vi "SHA-2_hash chunk_U32.vi"(0 "h in":u32[](array[numeric]), 1 "Chunk":u32[](array[numeric]), 12 "error in (no error)":errorcluster) -> (4 "h out":u32[](array[numeric]), 14 "error out":errorcluster)   [LabVIEW 2011, in "i3-external-encryption.lvlib"]
doc: "Hashes a U32 chunk.\n\n(c) Ton Plomp, 2011\nTHIS SOFTWARE IS PROVIDED AS IS, AND ANY WARRANTY IS REJECTED"
uses:
  i3-external-encryption.lvlib
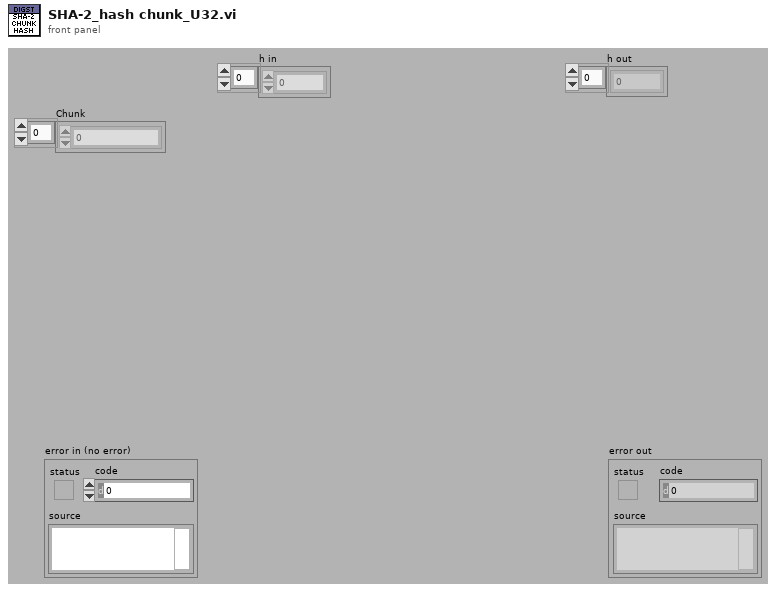
[diagram p1: front panel]
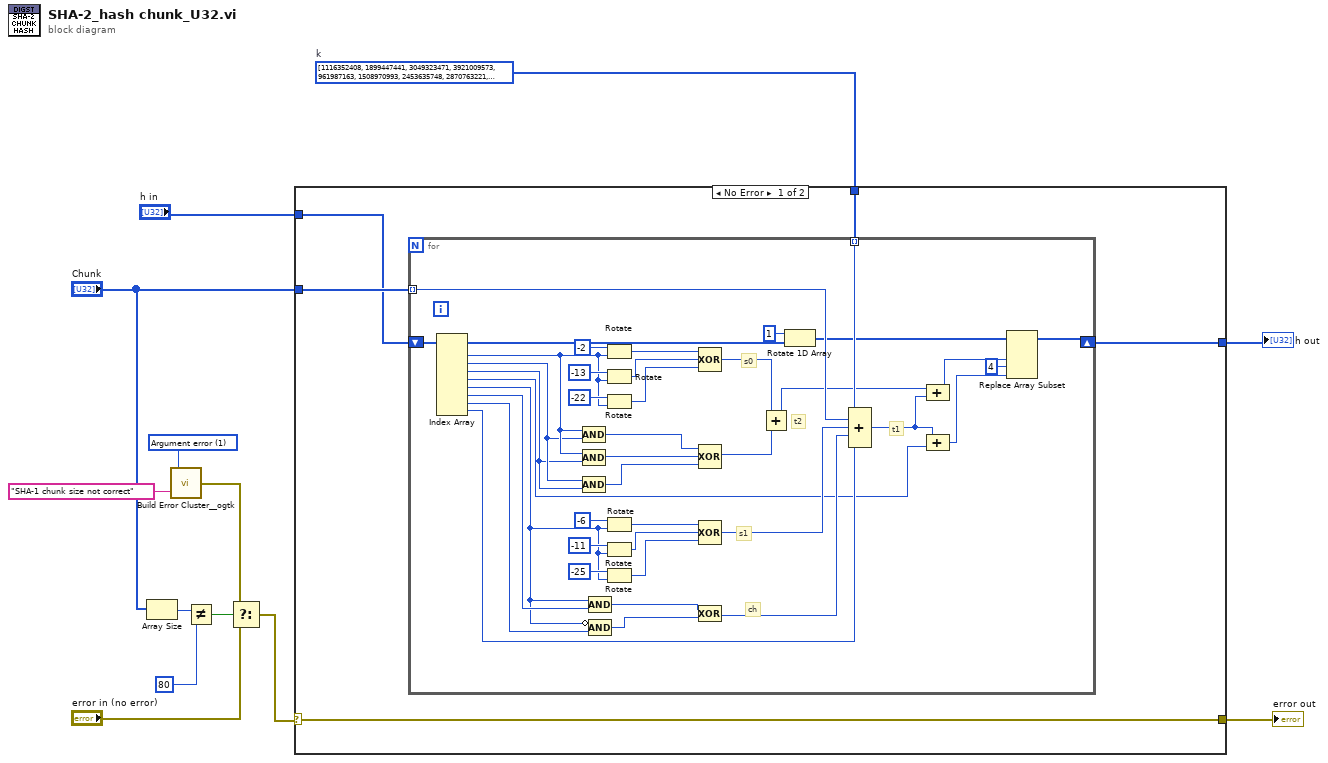
[diagram p0: block diagram]
diagram:
  w1 = u32[] [1116352408, 1899447441, 3049323471, 3921009573, 961987163, 1508970993, 2453635748, 2870763221, 3624381080, 310598401, 607225278, 1426881987, 1925078388, 2162078206, 2614888103, 3248222580, 3835390401, 4022224774, 264347078, 604807628, 770255983, 1249150122, 1555081692, 1996064986, 2554220882, 2821834349, 2952996808, 3210313671, 3336571891, 3584528711, 113926993, 338241895, 666307205, 773529912, 1294757372, 1396182291, 1695183700, 1986661051, 2177026350, 2456956037, 2730485921, 2820302411, 3259730800, 3345764771, 3516065817, 3600352804, 4094571909, 275423344, 430227734, 506948616, 659060556, 883997877, 958139571, 1322822218, 1537002063, 1747873779, 1955562222, 2024104815, 2227730452, 2361852424, 2428436474, 2756734187, 3204031479, 3329325298]  # k
  w4 = 1 items=["No error", "Argument error", "Memory is full", "Out of zone", "End of file", "File already open", "Generic file I/O error", "File not found", "File permission error", "Disk is full", "Duplicate path", "Too many files open", "System feature not enabled", "Resource file not found", "Cannot add resource", "Resource not found", "Image not found", "Image memory error", "Pen does not exist", "Config type invalid", "Config token not found", "Config parse error", "Config memory error", "Bad external code format", "Bad external code offset", "External code not present", "Null window", "Destroy window error", "Null menu", "Print aborted", "Bad print record", "Print driver error", "Windows error during printing", "Memory error during printing", "Print dialog error", "Generic print error", "Invalid device refnum", "Device not found", "Device parameter error", "Device unit error", "Cannot open device", "Device call aborted", "Generic error", "Cancelled by user", "Object ID too low", "Object ID too high", "Object not in heap", "Unknown heap", "Unknown object (invalid DefProc)", "Unknown object (DefProc not in table)", "Message out of range", "Invalid (null) method", "Unknown message", "Manager call not supported", "Bad address", "Network operation in progress", "Network operation timed out", "Connection is busy", "Network attribute not supported", "Network error", "Address in use", "System out of memory", "Connection aborted", "Connection refused", "Not connected", "Already connected", "Connection closed", "Initialization error (interapplication manager)", "Bad occurrence", "Wait on unbound occurrence handler", "Occurrence queue overflow", "Datalog type conflict", "Unused", "Unrecognized type (interapplication manager)", "Memory corrupt", "Failed to make temporary DLL", "Old CIN version", "Drag socket not found", "Failed to load drop-object", "Failed to register OLE object", "Failed to release OLE object", "Format specifier type mismatch", "Unknown format specifier", "Too few format specifiers", "Too many format specifiers", "Scan failed", "Newer CIN version", "Error converting to variant", "Runtime menu error", "Password tampered", "Variant attribute not found", "Incompatible variant data type", "Event data is not available", "Event Store is not present", "Occurrence is not found", "Event Queue is not created", "Event info is not available", "Refnum passed is NULL", "Error retrieving Class GUID", "Error retrieving CoClass GUID", "Error retrieving TypeLib GUID.", "Bad built application magic bytes.", "Specific driver is different from the specific driver associated with the Logical Name.", "There is no session opened to the class driver.", "Max Error", "MAX - Error with config objects", "MAX - Error loading configuration", "MAX - Group not supported"]
  n1 = Array Size(array="Chunk") -> (size(s)=w12:i32)
  n2 = call <userlib>:"Build Error Cluster__ogtk.vi"("String to Prepend to source (\"\")"="SHA-1 chunk size not correct" ("String to Prepend to source (\"\")"), "code"=w4) -> ("error out"=w6:errorcluster)
  n3 = Not Equal?(x=w12, y=80) -> (x != y?=w10:bool)
  n4 = Select(t=w6, s=w10, f="error in (no error)") -> (s? t:f=w8:errorcluster)
  n5 = case shown="No Error" w8 {
    selector: w8 -> [w17 w59]
    tunnel: "Chunk" -> [w18 _]
    tunnel: [w17 w59] -> w7
    tunnel: [w16 _] -> w3
    tunnel: "h in" -> [w15 _]
    tunnel: w1 -> [w14 _]
    frame No Error {
      n6 = for {
        tunnel: w18 -> [w30] mode=indexing
        shift-right: [w25] -> w16
        shift-left: w15 -> [w28]
        tunnel: w14 -> [w31] mode=indexing
        # "t1"
        # "ch"
        # "s1"
        # "t2"
        # "s0"
        n7 = Index Array(array=w28) -> (element #1=w52:u32, element #2=w51:u32, element #3=w50:u32, element #4=w24:u32, element #5=w37:u32, element #6=w38:u32, element #7=w36:u32, element #8=w29:u32)  [unwired: 8 in]
        n8 = Compound Arithmetic op=AND(w52, w51) -> (w49:u32)
        n9 = Compound Arithmetic op=AND(w52, w50) -> (w48:u32)
        n10 = Compound Arithmetic op=AND(w51, w50) -> (w47:u32)
        n11 = Compound Arithmetic op=AND(w37, w38) -> (w35:u32)
        n12 = Compound Arithmetic op=AND(invert w37, w36) -> (w34:u32)
        n13 = Rotate(1:w52, 2:i8 -2 ("y")) -> (0:w57:u32)
        n14 = Rotate(1:w52, 2:i8 -13 ("y")) -> (0:w55:u32)
        n15 = Rotate(1:w52, 2:i8 -22 ("y")) -> (0:w53:u32)
        n16 = Rotate(1:w37, 2:i8 -6 ("y")) -> (0:w42:u32)
        n17 = Rotate(1:w37, 2:i8 -11 ("y")) -> (0:w44:u32)
        n18 = Rotate(1:w37, 2:i8 -25 ("y")) -> (0:w46:u32)
        n19 = Compound Arithmetic op=XOR(w57, w55, w53) -> (w40:u32)
        n20 = Compound Arithmetic op=XOR(w49, w48, w47) -> (w39:u32)
        n21 = Compound Arithmetic op=XOR(w42, w44, w46) -> (w33:u32)
        n22 = Compound Arithmetic op=XOR(w35, w34) -> (w32:u32)
        n23 = Add(x=w40, y=w39) -> (x+y=w21:u32)
        n24 = Rotate 1D Array(1:w28, 2:1 ("n")) -> (0:w26:u32[])
        n25 = Compound Arithmetic op=ADD(w31, w30, w33, w32, w29) -> (w20:u32)
        n26 = Compound Arithmetic op=ADD(w21, w20) -> (w19:u32)
        n27 = Compound Arithmetic op=ADD(w20, w24) -> (w23:u32)
        n28 = Replace Array Subset(array=w26, new element #1=w19, new element #2=w23, index #2=4 ("index")) -> (w25:u32[])  [unwired: 1 in]
      }
    }
    frame Error {
    }
  }
  "error out" <- w7
  "h out" <- w3
